vi "Map from Monkeys' Notes.vi"(0 "Puzzle Input":string="        ...#\n        .#..\n        #...\n        ....\n...#.......#\n........#...\n..#....#....\n..........#.\n        ...#....\n        .....#..\n        .#......\n        ......#.\n\n10R5L5R10L4R5L5") -> (1 "Steps":T2[](array[typedef]), 2 "Board Map":T1[][](array[typedef]) items=["Empty", "Portal", "Open", "Wall", ">", "<", ">-^", ">-v", "^-<", "v-<"])   [LabVIEW 2020, in "AoC 2022.lvlib"]
uses:
  AoC 2022.lvlib
  Map Action.ctl
  Map Direction.ctl
  Map Action Step.ctl
  Map Tile.ctl
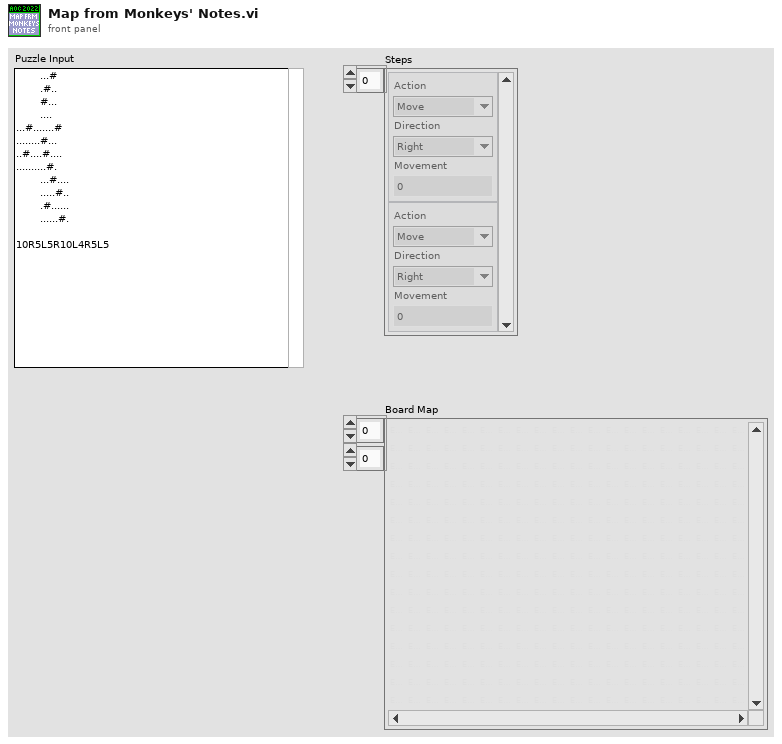
[diagram p1: front panel]
types:
  T1 = typedef "AoC 2022.lvlib/Map Tile.ctl" = u16
  T2 = typedef "AoC 2022.lvlib/Map Action Step.ctl" = cluster{"Action":T3, "Direction":T4, "Movement":i32}
  T3 = typedef "AoC 2022.lvlib/Map Action.ctl" = enum16{"Move", "Turn"}
  T4 = typedef "AoC 2022.lvlib/Map Direction.ctl" = enum16{"Facing", "Right", "Left", "Up", "Down"}
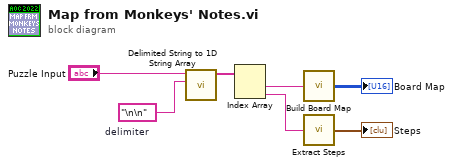
[diagram p0: block diagram]
diagram:
  w6 = "\n\n"  # delimiter
  n1 = call <vilib>:"Delimited String to 1D String Array.vi"("delimiter"=w6, "delimited string"="Puzzle Input") -> ("string array"=w5:string[])  [unwired: 9 in]
  n2 = Index Array(array=w5) -> (element #1=w4:string, element #2=w3:string)  [unwired: 2 in]
  n3 = call "Build Board Map.vi"("Map"=w4) -> ("Board Map"=→"Board Map":T1[][])
  n4 = call "Extract Steps.vi"("Instructions"=w3) -> ("Steps"=→"Steps":T2[])
